vi "example_05_create_graph.vi"() -> ()   [LabVIEW 2015, in "lv-graph.lvlib"]
doc: "Create graph shows how to generate data, store it in a graph, create an image of the graph and store it as a file."
uses:
  lv-graph.lvlib
  public/_controls/configuration_create_graph.ctl
  public/advanced/build_graph-single_axis.vi
panel:
  in  "configuration":T1={"X/Y Scales to Copy"=1, "Copy Graph Format?"=FALSE}
  in  "data_rate_ms":u32=10
  out "graph":T2(graph)
  in  "type":enum16{"Null", "PNG", "BMP", "JPEG"}(ring)=enum."PNG"
  in  "data_to_generate":i32=1000
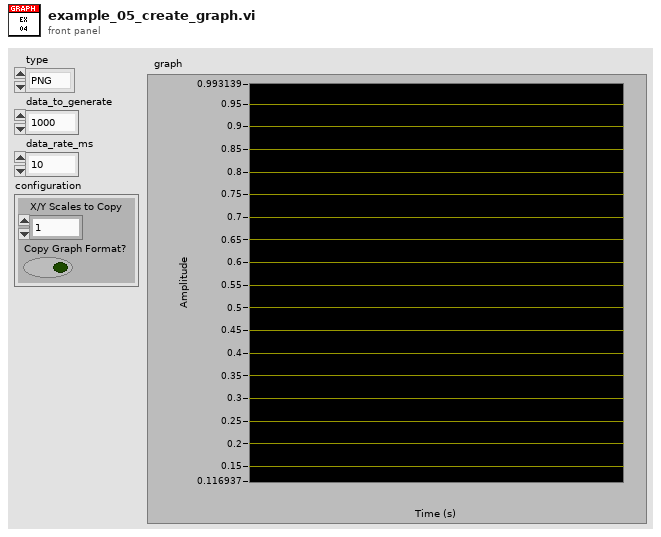
[diagram p1: front panel]
types:
  T1 = typedef "lv-graph.lvlib/configuration_create_graph.ctl" = cluster{"X/Y Scales to Copy":i32, "Copy Graph Format?":bool}
  T2 = cluster{"Time [] out":dbl[], "Data[][] out":dbl[]}[]
  T3 = cluster{"x_scale_maximum":dbl, "x_scale_minimum":dbl, "y_scale_maximum":dbl, "y_scale_minimum":dbl}
  T4 = typedef "imagedata.ctl" = cluster{"image type":i32, "image depth":i32, "image":u8[], "mask":u8[], "colors":u32[], "Rectangle":cluster{"left":i16, "top":i16, "right":i16, "bottom":i16}}
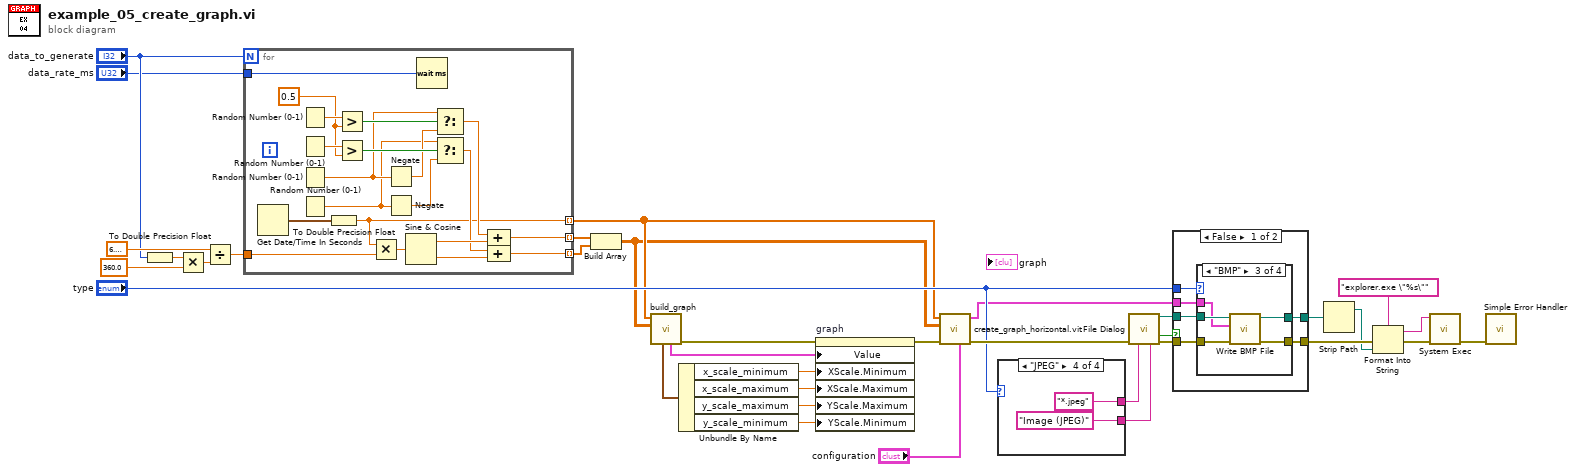
[diagram p0: block diagram]
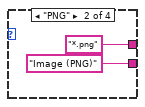
[diagram p3: hidden frame]
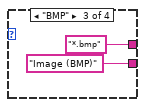
[diagram p4: hidden frame]
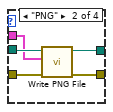
[diagram p6: hidden frame]
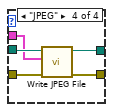
[diagram p7: hidden frame]
diagram:
  n1 = To Double Precision Float(number="data_to_generate") -> (double precision float=w31:dbl)
  n2 = Multiply(x=w31, y=360.0) -> (x*y=w32:dbl)
  n3 = Divide(x=6.283185307179586, y=w32) -> (x/y=w33:dbl)
  n4 = for {
    N: "data_to_generate" -> [_]
    tunnel: w33 -> [w55]
    tunnel: [w40] -> w2 mode=indexing
    tunnel: "data_rate_ms" -> [w39]
    tunnel: [w37] -> w7 mode=indexing
    tunnel: [w36] -> w6 mode=indexing
    w51 = 0.5 ("y")
    n5 = Get Date/Time In Seconds() -> (seconds since 1Jan1904=w38:timestamp)
    n6 = Random Number (0-1)() -> (number: 0 to 1=w53:dbl)
    n7 = Random Number (0-1)() -> (number: 0 to 1=w52:dbl)
    n8 = Random Number (0-1)() -> (number: 0 to 1=w48:dbl)
    n9 = Random Number (0-1)() -> (number: 0 to 1=w46:dbl)
    n10 = To Double Precision Float(number=w38) -> (double precision float=w40:dbl)
    n11 = Greater?(x=w53, y=w51) -> (0:w50:bool)
    n12 = Greater?(x=w52, y=w51) -> (0:w49:bool)
    n13 = Multiply(x=w40, y=w55) -> (x*y=w54:dbl)
    n14 = Negate(x=w48) -> (-x=w47:dbl)
    n15 = Negate(x=w46) -> (-x=w45:dbl)
    n16 = Sine & Cosine(0:w54) -> (1:w43:dbl, 2:w44:dbl)
    n17 = Wait (ms)(milliseconds to wait=w39) -> ()  [unwired: 1 out]
    n18 = Select(t=w48, s=w50, f=w47) -> (s? t:f=w42:dbl)
    n19 = Select(t=w46, s=w49, f=w45) -> (s? t:f=w41:dbl)
    n20 = Compound Arithmetic op=ADD(w42, w43) -> (w37:dbl)
    n21 = Compound Arithmetic op=ADD(w41, w44) -> (w36:dbl)
  }
  n22 = Build Array(w7, w6) -> (w1:dbl[][])
  n23 = call-poly "build_graph.vi"("y_axis"=w1, "x_axis"=w2) -> ("error out"=w10:errorcluster, "graph_data"=w3:cluster{dbl[], dbl[]}[], "scale_ranges"=w4:T3)  [unwired: 7 in]
  n24 = Unbundle By Name(w4) -> ("x_scale_minimum"=w12:dbl, "x_scale_maximum"=w11:dbl, "y_scale_maximum"=w13:dbl, "y_scale_minimum"=w14:dbl)
  n25 = property on="graph" class="XYGraph (strict)"(error in=w10, "Value"=w3, "XScale.Minimum"=w12, "XScale.Maximum"=w11, "YScale.Maximum"=w13, "YScale.Minimum"=w14) -> (error out=w9:errorcluster)  [unwired: 1 in, 1 out]
  n26 = call "create_graph_horizontal.vit"("configuration"="configuration", "error in"=w9, "y_axis"=w1, "x_axis"=w2) -> ("error out"=w26:errorcluster, "image_data"=w22:T4)  [unwired: 6 in]
  n27 = case shown="\"JPEG\"" "type" {
    tunnel: [_ "*.png" "*.bmp" "*.jpeg"] -> w24
    tunnel: [_ "Image (PNG)" "Image (BMP)" "Image (JPEG)"] -> w23
    frame Default {
    }
    frame "PNG" {
    }
    frame "BMP" {
    }
    frame "JPEG" {
    }
  }
  n28 = call "File Dialog"("error in"=w26, "pattern (all files)"=w24, "pattern label"=w23) -> ("selected path"=w27:path, "cancelled"=w28:bool, "error out"=w29:errorcluster)  [unwired: 9 in, 1 out]
  n29 = case shown="False" w28 {
    tunnel: "type" -> [w67 _]
    tunnel: w29 -> [w65 w84]
    tunnel: [w66 w84] -> w20
    tunnel: w27 -> [w64 _]
    tunnel: w22 -> [w63 _]
    tunnel: [w62 _] -> w21
    frame False {
      n30 = case shown="\"BMP\"" w67 {
        tunnel: [w68 w72 w77 w82] -> w66
        tunnel: w65 -> [w68 w73 w78 w83]
        tunnel: w64 -> [_ w71 w76 w81]
        tunnel: w63 -> [_ w70 w75 w80]
        tunnel: [_ w69 w74 w79] -> w62
        frame Default {
        }
        frame "PNG" {
          n31 = call <vilib>:"Write PNG File.vi"("error in (no error)"=w73, "image data"=w70, "path to PNG file"=w71) -> ("error out"=w72:errorcluster, "path"=w69:path)  [unwired: 7 in]
        }
        frame "BMP" {
          n32 = call <vilib>:"Write BMP File.vi"("error in (no error)"=w78, "image data"=w75, "path to BMP file"=w76) -> ("error out"=w77:errorcluster, "path"=w74:path)  [unwired: 7 in]
        }
        frame "JPEG" {
          n33 = call <vilib>:"Write JPEG File.vi"("error in (no error)"=w83, "image data"=w80, "path to JPEG file"=w81) -> ("error out"=w82:errorcluster, "path"=w79:path)  [unwired: 7 in]
        }
      }
    }
    frame True {
    }
  }
  n34 = Strip Path(path=w21) -> (stripped path=w19:path)  [unwired: 1 out]
  n35 = Format Into String(format string="explorer.exe \"%s\"", error in=w20, w19) -> (resulting string=w16:string, error out=w17:errorcluster)  [unwired: 1 in]
  n36 = call <vilib>:"System Exec.vi"("error in (no error)"=w17, "command line"=w16) -> ("error out"=w15:errorcluster)  [unwired: 6 in, 3 out]
  n37 = call <vilib>:"Simple Error Handler.vi"("error in (no error)"=w15) -> ()  [unwired: 4 in, 5 out]
